vi "Disconnect Clock Terminals-Array.vi"(8 "error in (no error)":errorcluster, 10 "Clock Routing":T1[](array[typedef]), 11 "instrument handle":refnum<k15>) -> (0 "error out":errorcluster, 3 "instrument handle out":refnum<k15>)   [LabVIEW 2026]
doc: "Allow for cluster input containing clock source and destination information. Uses the NI-SYNC driver to disconnects the clocks."
uses:
  Clock Routing.ctl
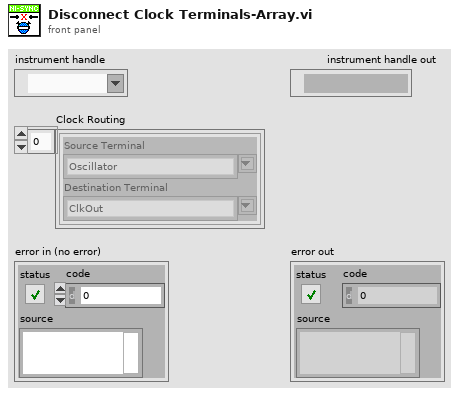
[diagram p1: front panel]
types:
  T1 = typedef "Clock Routing.ctl" = cluster{"Source Terminal":string, "Destination Terminal":string}
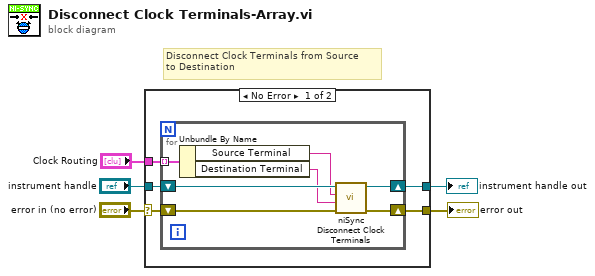
[diagram p0: block diagram]
diagram:
  # "Disconnect Clock Terminals from Source\nto Destination"
  n1 = case shown="No Error" "error in (no error)" {
    selector: "error in (no error)" -> [w8 w19]
    tunnel: "instrument handle" -> [w10 w18]
    tunnel: [w9 w18] -> w4
    tunnel: [w7 w19] -> w2
    tunnel: "Clock Routing" -> [w6 _]
    frame No Error {
      n2 = for {
        tunnel: w6 -> [w13] mode=indexing
        shift-right: [w16] -> w9
        shift-left: w10 -> [w17]
        shift-right: [w14] -> w7
        shift-left: w8 -> [w15]
        n3 = Unbundle By Name(w13) -> ("Source Terminal"=w12:string, "Destination Terminal"=w11:string)
        n4 = call <instrlib>:"niSync Disconnect Clock Terminals.vi"("error in (no error)"=w15, "destination terminal"=w11, "source terminal"=w12, "instrument handle"=w17) -> ("error out"=w14:errorcluster, "instrument handle out"=w16:refnum<k15>)  [unwired: 6 in]
      }
    }
    frame Error {
    }
  }
  "instrument handle out" <- w4
  "error out" <- w2
